vi "Size Grove to Smalles Rectangle.vi"(11 "Grove":T1[][](array[typedef])) -> (3 "Sized Grove":T1[][](array[typedef]))   [LabVIEW 2020]
uses:
  RB ENUM_Spot ID.ctl
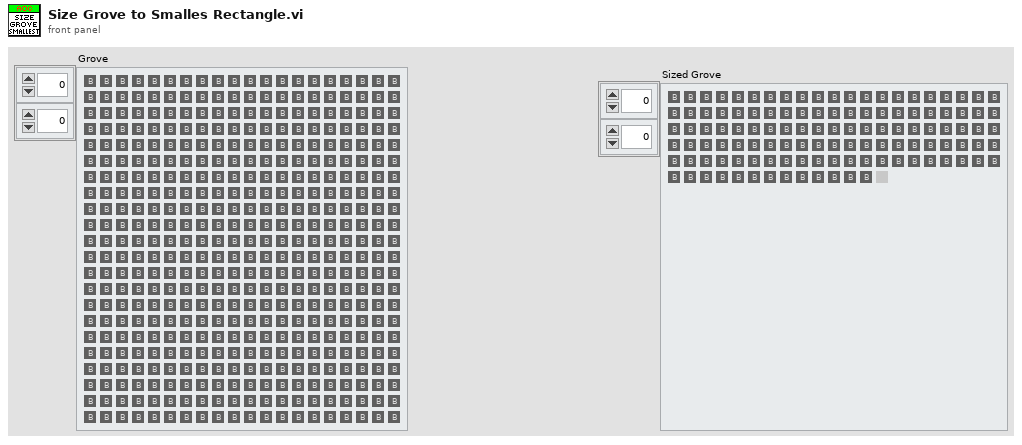
[diagram p1: front panel]
types:
  T1 = typedef "RB ENUM_Spot ID.ctl" = enum32{"Blank", "ELF", "Proposed"}
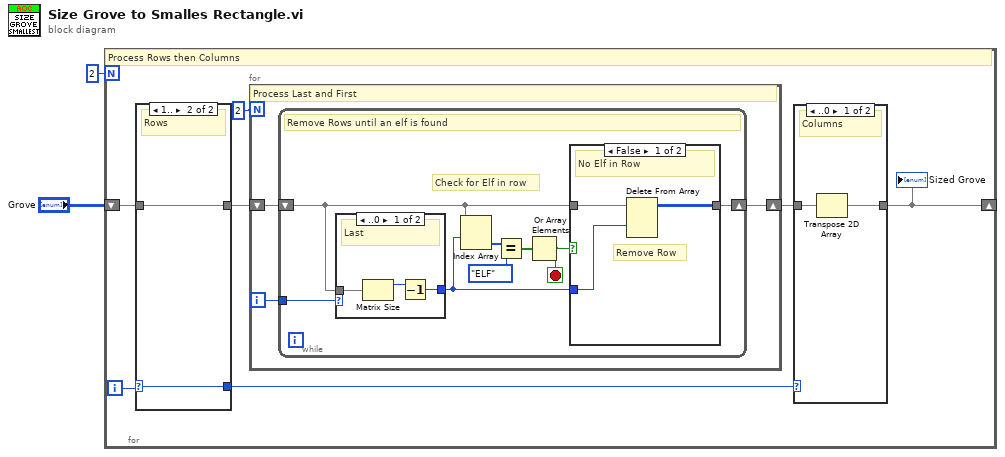
[diagram p0: block diagram]
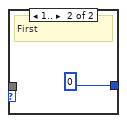
[diagram p3: hidden frame]
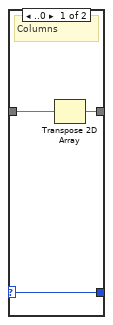
[diagram p5: hidden frame]
diagram:
  n1 = for {
    N: 2 -> [_]
    shift-right: [w3] -> _
    shift-left: "Grove" -> [w8]
    i -> [w9]
    # "Process Rows then Columns"
    n2 = case shown="1.." w9 {
      selector: w9 -> [w34 w35]
      tunnel: [w34 w35] -> w7
      tunnel: w8 -> [w33 w36]
      tunnel: [w32 w36] -> w6
      frame ..0 {
        # "Columns"
        n3 = Transpose 2D Array(2D array=w33) -> (transposed array=w32:T1[][])
      }
      frame 1.. {
        # "Rows"
      }
    }
    n4 = for {
      N: 2 -> [_]
      shift-right: [w10] -> w5
      shift-left: w6 -> [w11]
      i -> [w12]
      # "Process Last and First"
      n5 = while {
        tunnel: w12 -> [w20]
        shift-right: [w15] -> w10
        shift-left: w11 -> [w16]
        stop <- w14 stop-if-true
        # "Check for Elf in row"
        # "Remove Rows until an elf is found"
        n6 = case shown="..0" w20 {
          tunnel: [w25 0 ("index (row)")] -> w13
          tunnel: w16 -> [w27 _]
          frame ..0 {
            # "Last"
            n7 = Matrix Size(0:w27) -> (1:w26:i32)  [unwired: 1 out]
            n8 = Decrement(x=w26) -> (x-1=w25:i32)
          }
          frame 1.. {
            # "First"
          }
        }
        n9 = Index Array(array=w16, index (row)=w13) -> (element=w19:T1[])  [unwired: 1 in]
        n10 = Equal?(x=w19, y=RB_ENUM_Spot_ID."ELF" ("Spot")) -> (x = y?=w17:bool[])
        n11 = Or Array Elements(Boolean array=w17) -> (logical OR=w14:bool)
        n12 = case shown="False" w14 {
          tunnel: w16 -> [w23 w24]
          tunnel: [w22 w24] -> w15
          tunnel: w13 -> [w21 _]
          frame False {
            # "Remove Row"
            # "No Elf in Row"
            n13 = Delete From Array(array=w23, index (row)=w21) -> (array with subset deleted=w22:T1[][])  [unwired: 2 in, 1 out]
          }
          frame True {
            # "Leave As is"
            # "Elf in Row"
          }
        }
      }
    }
    n14 = case shown="..0" w7 {
      tunnel: w5 -> [w30 w31]
      tunnel: [w29 w31] -> w3
      frame ..0 {
        # "Columns"
        n15 = Transpose 2D Array(2D array=w30) -> (transposed array=w29:T1[][])
      }
      frame 1.. {
        # "Rows"
      }
    }
    "Sized Grove" <- w3
  }
